vi "Insert Image.vi"() -> ()   [LabVIEW 2016]
panel:
  in  "Picture Type":enum16{"BMP", "JPG", "PNG"}(ring)
  in  "Picture File Path":path
  out "new picture":picture
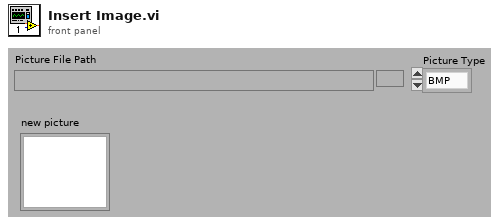
[diagram p1: front panel]
types:
  T1 = typedef "imagedata.ctl" = cluster{"image type":i32, "image depth":i32, "image":u8[], "mask":u8[], "colors":u32[], "Rectangle":cluster{"left":i16, "top":i16, "right":i16, "bottom":i16}}
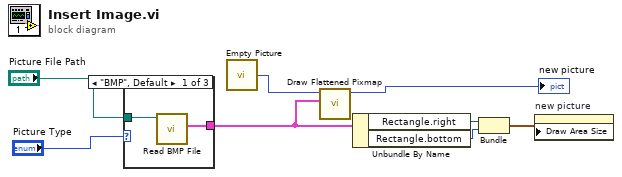
[diagram p0: block diagram]
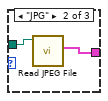
[diagram p2: hidden frame]
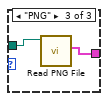
[diagram p3: hidden frame]
diagram:
  n1 = case shown="\"BMP\", Default" "Picture Type" {
    tunnel: "Picture File Path" -> [w10 w11 w13]
    tunnel: [w9 w12 w14] -> w5
    frame "BMP", Default {
      n2 = call <vilib>:"Read BMP File.vi"("path to BMP file"=w10) -> ("image data"=w9:T1)  [unwired: 8 in, 2 out]
    }
    frame "JPG" {
      n3 = call <vilib>:"Read JPEG File.vi"("path to JPEG file"=w11) -> ("image data"=w12:T1)  [unwired: 8 in, 2 out]
    }
    frame "PNG" {
      n4 = call <vilib>:"Read PNG File.vi"("path to PNG file"=w13) -> ("image data"=w14:T1)  [unwired: 8 in, 2 out]
    }
  }
  n5 = call "Empty Picture"() -> ("empty picture"=w8:picture)
  n6 = call <vilib>:"Draw Flattened Pixmap.vi"("image data"=w5, "picture"=w8) -> ("new picture"=→"new picture":picture)  [unwired: 7 in]
  n7 = Unbundle By Name(w5) -> ("Rectangle.right"=w4:i16, "Rectangle.bottom"=w3:i16)
  n8 = Bundle("right"=w4, "bottom"=w3) -> (w2:cluster{"right":i16, "bottom":i16})  [unwired: 1 in]
  n9 = property on="new picture" class="Pict"("Draw Area Size"=w2) -> ()  [unwired: 2 in, 2 out]
